vi "字符串与实际变量转换-状态参数.vi"(4 "状态参数":string[](array[string])) -> ()   [LabVIEW 2013]
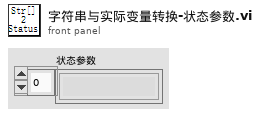
[diagram p1: front panel]
types:
  T1 = cluster{"联机状态":bool, "外置清零信号":bool, "卡件工作模式":enum16{"无输出", "正常工作", "阀门常开", "阀门常闭"}, "卡件序列号":string, "卡件物理地址":string, "伺服阀输出电流CH1":dbl, "输出通道状态CH1":bool, "伺服阀输出电流CH2":dbl, "输出通道状态CH2":bool, "伺服输出使能CH1 ":bool, "伺服输出使能CH2":bool, "LVDT1类型":enum16{"未接入", "直流", "交流"}, "LVDT1直流回路":bool, "LVDT1次级线圈 2":bool, "LVDT1次级线圈 1":bool, "LVDT1初级线圈":bool, "LVDT2类型":enum16{"未接入", "直流", "交流"}, "LVDT2直流回路":bool, "LVDT2次级线圈 2":bool, "LVDT2次级线圈 1":bool, "LVDT2初级线圈":bool, "DEH回路状态":bool, "DEH类型":enum16{"内置", "外接"}, "转速反馈使能":bool, "LVDT1信号采样百分比":dbl, "LVDT2信号采样百分比":dbl, "DEH指令值":u8, "转速差反馈量":dbl, "回路1转速":dbl, "回路2转速":dbl, "回路3转速":dbl, "中选转速":dbl, "LVDT1 ADC":i16, "LVDT2 ADC":i16, "DEH ADC":i16, "LVDT1ZADC":i16, "LVDT2ZADC":i16, "LVDT1FADC":i16, "LVDT2FADC":i16, "DehZeroCali":bool, "DehFullCali":bool, "LVDT1ZeroCali":bool, "LVDT1FullCali":bool, "LVDT2ZeroCali":bool, "LVDT2FullCali":bool, "转速零度标定":i16, "转速满度标定":i16, "转速指令采样值":i16, "标准转速":dbl}
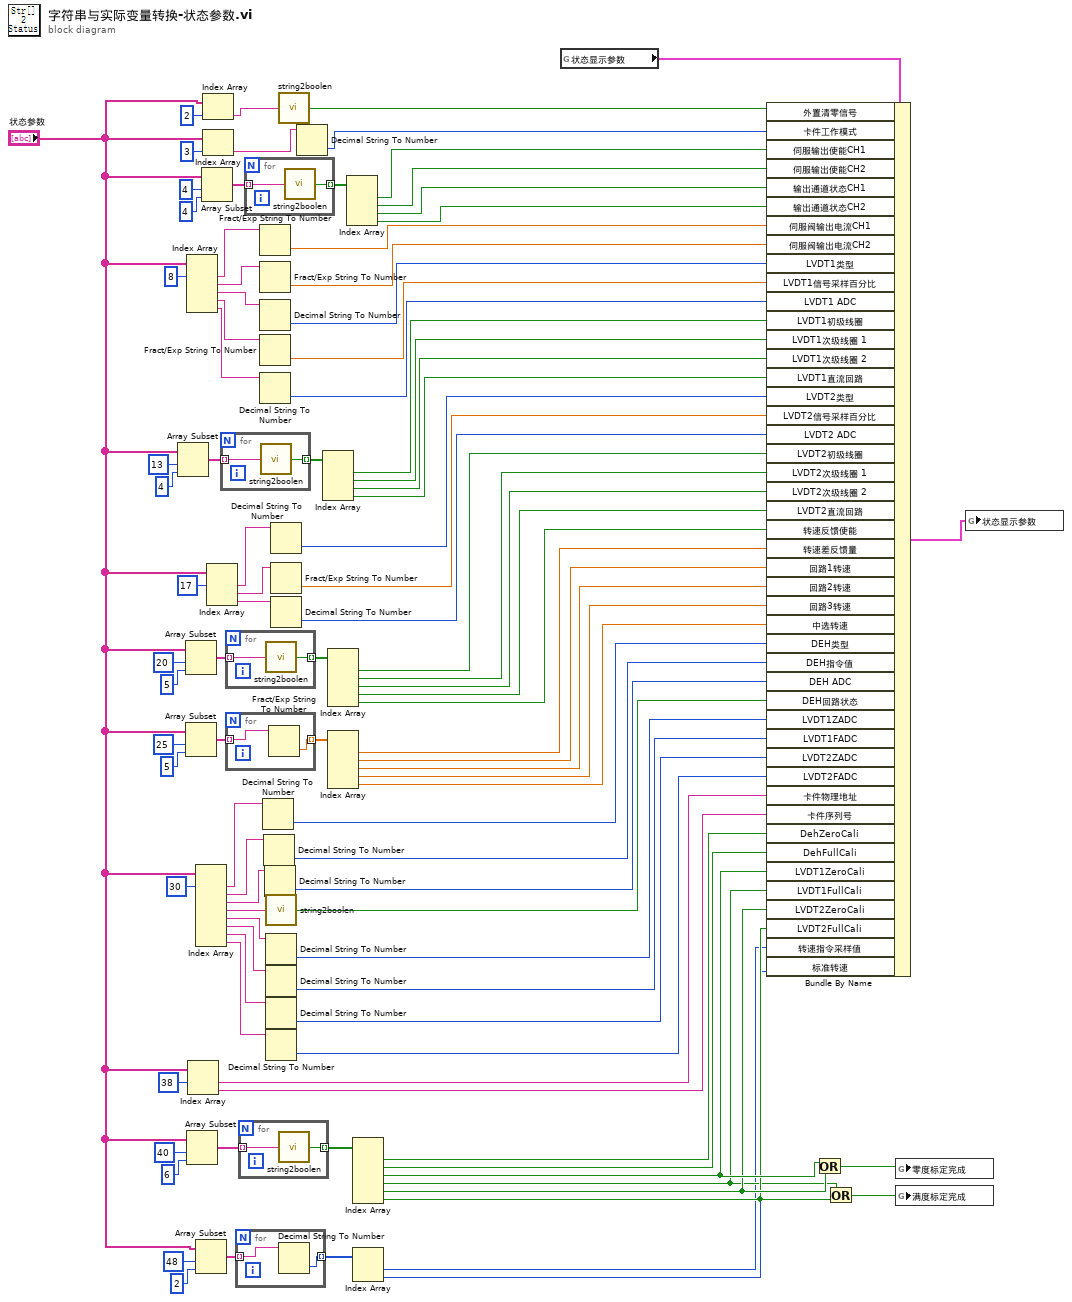
[diagram p0: block diagram]
diagram:
  n1 = Array Subset(array="状态参数", index=13, length=4) -> (w75:string[])
  n2 = Array Subset(array="状态参数", index=20, length=5) -> (w62:string[])
  n3 = Array Subset(array="状态参数", index=25, length=5) -> (w53:string[])
  n4 = Index Array(array="状态参数", index #1=8 ("index")) -> (element #1=w85:string, element #2=w83:string, element #3=w81:string, element #4=w79:string, element #5=w40:string)  [unwired: 4 in]
  n5 = Array Subset(array="状态参数", index=40, length=6) -> (w17:string[])
  n6 = Index Array(array="状态参数", index #1=38 ("index")) -> (element #1=w21:string, element #2=w20:string)  [unwired: 1 in]
  n7 = Index Array(array="状态参数", index #1=30 ("index")) -> (element #1=w45:string, element #2=w44:string, element #3=w37:string, element #4=w38:string, element #5=w30:string, element #6=w29:string, element #7=w28:string, element #8=w27:string)  [unwired: 7 in]
  n8 = Array Subset(array="状态参数", index=48, length=2) -> (w5:string[])
  n9 = Array Subset(array="状态参数", index=4, length=4) -> (w92:string[])
  n10 = Index Array(array="状态参数", index=2) -> (element=w32:string)
  n11 = Index Array(array="状态参数", index=3) -> (element=w96:string)
  n12 = Index Array(array="状态参数", index #1=17 ("index")) -> (element #1=w68:string, element #2=w66:string, element #3=w35:string)  [unwired: 2 in]
  n13 = for {
    tunnel: w75 -> [w101] mode=indexing
    tunnel: [w100] -> w74 mode=indexing
    n14 = call "string2boolen.vi"("String"=w101) -> ("Boolean"=w100:bool)
  }
  n15 = for {
    tunnel: w62 -> [w103] mode=indexing
    tunnel: [w102] -> w61 mode=indexing
    n16 = call "string2boolen.vi"("String"=w103) -> ("Boolean"=w102:bool)
  }
  n17 = for {
    tunnel: w53 -> [w105] mode=indexing
    tunnel: [w104] -> w52 mode=indexing
    n18 = Fract/Exp String To Number(string=w105) -> (number=w104:dbl)  [unwired: 3 in, 1 out]
  }
  n19 = for {
    tunnel: w5 -> [w107] mode=indexing
    tunnel: [w106] -> w3 mode=indexing
    n20 = Decimal String To Number(string=w107) -> (number=w106:i32)  [unwired: 2 in, 1 out]
  }
  n21 = for {
    tunnel: w17 -> [w109] mode=indexing
    tunnel: [w108] -> w16 mode=indexing
    n22 = call "string2boolen.vi"("String"=w109) -> ("Boolean"=w108:bool)
  }
  n23 = for {
    tunnel: w92 -> [w111] mode=indexing
    tunnel: [w110] -> w91 mode=indexing
    n24 = call "string2boolen.vi"("String"=w111) -> ("Boolean"=w110:bool)
  }
  n25 = Fract/Exp String To Number(string=w85) -> (number=w84:dbl)  [unwired: 3 in, 1 out]
  n26 = Fract/Exp String To Number(string=w83) -> (number=w82:dbl)  [unwired: 3 in, 1 out]
  n27 = Decimal String To Number(string=w81) -> (number=w80:i32)  [unwired: 2 in, 1 out]
  n28 = Fract/Exp String To Number(string=w79) -> (number=w78:dbl)  [unwired: 3 in, 1 out]
  n29 = Decimal String To Number(string=w40) -> (number=w39:i32)  [unwired: 2 in, 1 out]
  n30 = Decimal String To Number(string=w45) -> (number=w42:i32)  [unwired: 2 in, 1 out]
  n31 = Decimal String To Number(string=w44) -> (number=w43:i32)  [unwired: 2 in, 1 out]
  n32 = Decimal String To Number(string=w37) -> (number=w36:i32)  [unwired: 2 in, 1 out]
  n33 = call "string2boolen.vi"("String"=w38) -> ("Boolean"=w41:bool)
  n34 = Decimal String To Number(string=w30) -> (number=w26:i32)  [unwired: 2 in, 1 out]
  n35 = Decimal String To Number(string=w29) -> (number=w23:i32)  [unwired: 2 in, 1 out]
  n36 = Decimal String To Number(string=w28) -> (number=w24:i32)  [unwired: 2 in, 1 out]
  n37 = Decimal String To Number(string=w27) -> (number=w25:i32)  [unwired: 2 in, 1 out]
  n38 = Decimal String To Number(string=w68) -> (number=w67:i32)  [unwired: 2 in, 1 out]
  n39 = Fract/Exp String To Number(string=w66) -> (number=w65:dbl)  [unwired: 3 in, 1 out]
  n40 = Decimal String To Number(string=w35) -> (number=w34:i32)  [unwired: 2 in, 1 out]
  n41 = call "string2boolen.vi"("String"=w32) -> ("Boolean"=w31:bool)
  n42 = Decimal String To Number(string=w96) -> (number=w95:i32)  [unwired: 2 in, 1 out]
  n43 = Index Array(array=w74) -> (element #1=w73:bool, element #2=w72:bool, element #3=w71:bool, element #4=w70:bool)  [unwired: 4 in]
  n44 = Index Array(array=w61) -> (element #1=w60:bool, element #2=w59:bool, element #3=w58:bool, element #4=w57:bool, element #5=w56:bool)  [unwired: 5 in]
  n45 = Index Array(array=w52) -> (element #1=w51:dbl, element #2=w50:dbl, element #3=w49:dbl, element #4=w48:dbl, element #5=w47:dbl)  [unwired: 5 in]
  n46 = Index Array(array=w91) -> (element #1=w90:bool, element #2=w89:bool, element #3=w88:bool, element #4=w87:bool)  [unwired: 4 in]
  n47 = Index Array(array=w16) -> (element #1=w15:bool, element #2=w14:bool, element #3=w13:bool, element #4=w9:bool, element #5=w12:bool, element #6=w10:bool)  [unwired: 6 in]
  n48 = Index Array(array=w3) -> (element #1=w2:i32, element #2=w1:i32)  [unwired: 2 in]
  n49 = global read "状态显示参数.vi" "状态显示参数"() -> (w99:T1)
  n50 = Bundle By Name(cluster=w99, "外置清零信号"=w31, "卡件工作模式"=w95, "伺服输出使能CH1"=w90, "伺服输出使能CH2"=w89, "输出通道状态CH1"=w88, "输出通道状态CH2"=w87, "伺服阀输出电流CH1"=w84, "伺服阀输出电流CH2"=w82, "LVDT1类型"=w80, "LVDT1信号采样百分比"=w78, "LVDT1 ADC"=w39, "LVDT1初级线圈"=w73, "LVDT1次级线圈 1"=w72, "LVDT1次级线圈 2"=w71, "LVDT1直流回路"=w70, "LVDT2类型"=w67, "LVDT2信号采样百分比"=w65, "LVDT2 ADC"=w34, "LVDT2初级线圈"=w60, "LVDT2次级线圈 1"=w59, "LVDT2次级线圈 2"=w58, "LVDT2直流回路"=w57, "转速反馈使能"=w56, "转速差反馈量"=w51, "回路1转速"=w50, "回路2转速"=w49, "回路3转速"=w48, "中选转速"=w47, "DEH类型"=w42, "DEH指令值"=w43, "DEH ADC"=w36, "DEH回路状态"=w41, "LVDT1ZADC"=w26, "LVDT1FADC"=w23, "LVDT2ZADC"=w24, "LVDT2FADC"=w25, "卡件物理地址"=w21, "卡件序列号"=w20, "DehZeroCali"=w15, "DehFullCali"=w14, "LVDT1ZeroCali"=w13, "LVDT1FullCali"=w9, "LVDT2ZeroCali"=w12, "LVDT2FullCali"=w10, "转速指令采样值"=w2, "标准转速"=w1) -> (w98:T1)
  n51 = Or(x=w13, y=w12) -> (x .or. y?=w11:bool)
  n52 = Or(x=w9, y=w10) -> (x .or. y?=w8:bool)
  n53 = global write "零度标定完成.vi" "零度标定完成"(w11) -> ()
  n54 = global write "满度标定完成.vi" "满度标定完成"(w8) -> ()
  n55 = global write "状态显示参数.vi" "状态显示参数"(w98) -> ()
